vi "Winch v3.vi"() -> ()   [LabVIEW 2013]
uses:
  <vilib>/Rock Robotics/WPI/Joystick/WPI_JoystickGetSetRefNum.vi
  Robot Global Data.vi
  Globals/Useful Values.vi
  Globals/Homes.vi
  <vilib>/addons/control/pid/pid.llb/PID (DBL).vi
  Globals/Data for Dashboard.vi
  <vilib>/Utility/file.llb/Write To Spreadsheet File (DBL).vi
  <vilib>/addons/control/pid/NI_PID_pid.lvlib
panel:
  in  "Pullback Speed":dbl=-1.0
  in  "PID gains":T1={"proportional gain (Kc)"=2.75, "integral time (Ti, min)"=0.0, "derivative time (Td, min)"=0.0} {"derivative time (Td, min)" format="%.3f"; "integral time (Ti, min)" format="%.3f"; "proportional gain (Kc)" format="%.3f"}
  # "PULLBACK SPEED NEEDS\nTO BE NEGATIVE OR ELSE"
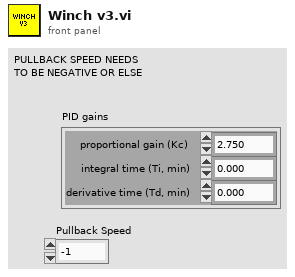
[diagram p1: front panel]
types:
  T1 = cluster{"proportional gain (Kc)":dbl, "integral time (Ti, min)":dbl, "derivative time (Td, min)":dbl}
  T2 = typedef "WPI_JoystickDevRef.ctl" = cluster{"Device":T3}
  T3 = typedef "WPI_JoystickDeviceEnum.ctl" = enum16{"USB 1", "USB 2", "USB 3", "USB 4", "Kinect 1", "Kinect 2"}
  T4 = typedef "WPI_MotorControlDeviceRef.ctl" = cluster{"DeviceStatus":errorcluster, "Type":enum16{"PWM", "CAN"}, "PWM":cluster{"Digital Module":T5, "PWM Channel":T6, "DeadBand":T7}, "CAN":cluster{"Device Number":u8, "Control Mode":T8, "Semaphore":T9, "Max Vout":dbl}, "Invert":bool, "TransformRef":T10, "InvTransformRef":T10}
  T5 = typedef "FPGA_TypedefDigitalModule.ctl" = enum16{"Digital Module 1", "Digital Module 2"}
  T6 = typedef "FPGA_DIOPWMChannel.ctl" = enum8{"PWM 1", "PWM 2", "PWM 3", "PWM 4", "PWM 5", "PWM 6", "PWM 7", "PWM 8", "PWM 9", "PWM 10", "Invalid"}
  T7 = typedef "WPI_PWMDeadband.ctl" = cluster{"Name":string, "maxPositivePwm":i32, "minPositivePwm":i32, "centerPwm":i32, "maxNegativePwm":i32, "minNegativePwm":i32, "angularRange":u16}
  T8 = typedef "WPI_CANJaguar_ControlMode.ctl" = enum8{"Percent VBus", "Current", "Speed", "Position", "Voltage"}
  T9 = typedef "Semaphore RefNum" = refnum<k1>
  T10 = typedef "WPI_PWMTransform_ConPane.ctl" = refnum<vi>
  T11 = typedef "WPI_AnalogChannelDevRef.ctl" = cluster{"DevStatus":errorcluster, "Analog Module":T12, "Analog Channel":T13}
  T12 = typedef "FPGA_TypedefAnalogModule.ctl" = enum16{"Analog Module 1", "Analog Module 2"}
  T13 = typedef "FPGA_AIChannel.ctl" = enum8{"AI 1", "AI 2", "AI 3", "AI 4", "AI 5", "AI 6", "AI 7", "AI 8", "Invalid"}
  T14 = typedef "WPI_DigitalInputDevRef.ctl" = cluster{"DevStatus":errorcluster, "DIO Channel":T15, "Digital Module":T5}
  T15 = typedef "FPGA_DIOChannel.ctl" = enum8{"DIO 1", "DIO 2", "DIO 3", "DIO 4", "DIO 5", "DIO 6", "DIO 7", "DIO 8", "DIO 9", "DIO 10", "DIO 11", "DIO 12", "DIO 13", "DIO 14", "Invalid"}
  T16 = typedef "WPI_DriverStationRobotMode2.ctl" = enum16{"Autonomous Disabled", "Autonomous Enabled", "Teleop Disabled", "Teleop Enabled", "Timeout", "Finish", "Test Disabled", "Test Enabled"}
  T17 = typedef "WPI_JoystickButtonState.ctl" = cluster{"Button 1":bool, "Button 2":bool, "Button 3":bool, "Button 4":bool, "Button 5":bool, "Button 6":bool, "Button 7":bool, "Button 8":bool, "Button 9":bool, "Button 10":bool, "Button 11":bool, "Button 12":bool}
  T18 = cluster{"axis 1 (x)":dbl, "axis 2 (y)":dbl, "axis 3 (throttle)":dbl, "axis 4":dbl, "axis 5":dbl, "axis 6":dbl}
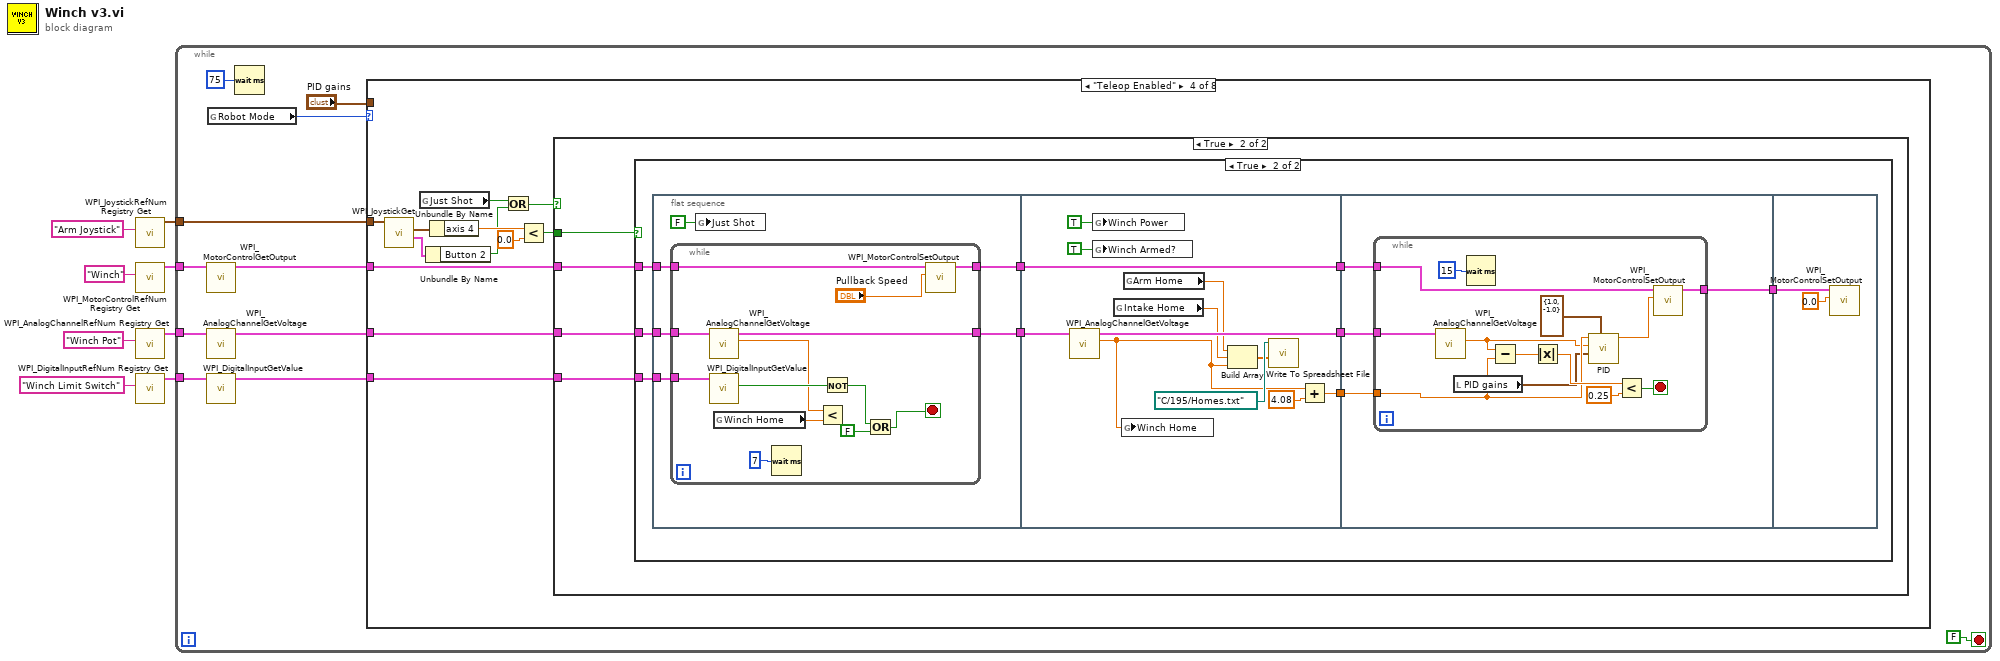
[diagram p0: block diagram]
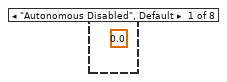
[diagram p2: hidden frame]
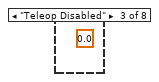
[diagram p4: hidden frame]
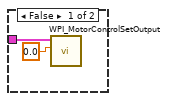
[diagram p5: hidden frame]
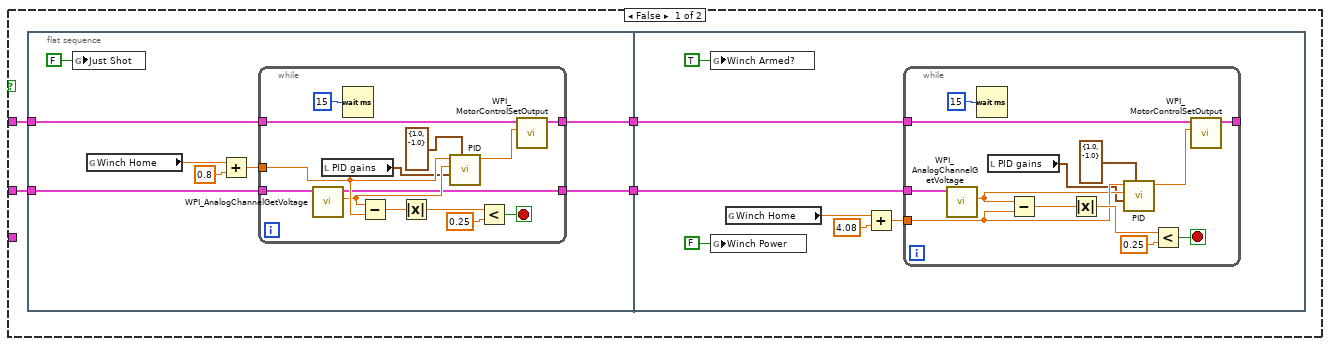
[diagram p6: hidden frame]
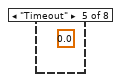
[diagram p7: hidden frame]
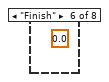
[diagram p8: hidden frame]
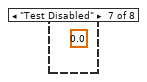
[diagram p9: hidden frame]
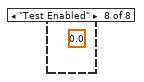
[diagram p10: hidden frame]
diagram:
  n1 = call <vilib>:"WPI_JoystickRefNum Registry Get.vi"("refnum name"="Arm Joystick") -> ("JoystickDevRef"=w3:T2)  [unwired: 9 in, 1 out]
  n2 = call <vilib>:"WPI_MotorControlRefNum Registry Get.vi"("refnum name"="Winch") -> ("MotorControlDevRef"=w5:T4)  [unwired: 9 in, 1 out]
  n3 = call <vilib>:"WPI_AnalogChannelRefNum Registry Get.vi"("refnum name"="Winch Pot") -> ("AIDeviceRef"=w8:T11)  [unwired: 9 in, 1 out]
  n4 = call <vilib>:"WPI_DigitalInputRefNum Registry Get.vi"("refnum name"="Winch Limit Switch") -> ("DigitalInputDevRef"=w2:T14)  [unwired: 9 in, 1 out]
  n5 = while {
    tunnel: w8 -> [w17]
    tunnel: w5 -> [w12]
    tunnel: w3 -> [w14]
    tunnel: w2 -> [w10]
    stop <- FALSE stop-if-true
    n6 = call <vilib>:"WPI_MotorControlGetOutput.vi"("MotorControlDevRef"=w12) -> ("MotorControlDevRef"=w11:T4)  [unwired: 8 in, 2 out]
    n7 = call <vilib>:"WPI_AnalogChannelGetVoltage.vi"("AIDeviceRef"=w17) -> ("AIDeviceRef"=w13:T11)  [unwired: 8 in, 2 out]
    n8 = call <vilib>:"WPI_DigitalInputGetValue.vi"("DigitalInputDevRef"=w10) -> ("DigitalInputDevRef"=w9:T14)  [unwired: 8 in, 2 out]
    n9 = global read "Robot Global Data.vi" "Robot Mode"() -> (w16:T16)
    n10 = Wait (ms)(milliseconds to wait=u32 75) -> ()  [unwired: 1 out]
    n11 = case shown="\"Teleop Enabled\"" w16 {
      tunnel: w11 -> [_ _ _ w28 _ _ _ _]
      tunnel: "PID gains" -> [_ _ _ _ _ _ _ _]
      tunnel: w14 -> [_ _ _ w31 _ _ _ _]
      tunnel: w9 -> [_ _ _ w29 _ _ _ _]
      tunnel: w13 -> [_ _ _ w27 _ _ _ _]
      frame "Autonomous Disabled", Default {
        (unwired) 0.0 ("Motor Output")
      }
      frame "Autonomous Enabled" {
      }
      frame "Teleop Disabled" {
        (unwired) 0.0 ("Motor Output")
      }
      frame "Teleop Enabled" {
        n12 = call <vilib>:"WPI_JoystickGet.vi"("JoystickDevRef"=w31) -> ("Buttons"=w30:T17, "Axes"=w26:T18)  [unwired: 4 in, 1 out]
        n13 = global read "Useful Values.vi" "Just Shot"() -> (w22:bool)
        n14 = Unbundle By Name(w30) -> ("Button 2"=w21:bool)
        n15 = Unbundle By Name(w26) -> ("axis 4"=w25:dbl)
        n16 = Or(x=w22, y=w21) -> (x .or. y?=w20:bool)
        n17 = Less?(x=w25, y=0.0) -> (x < y?=w23:bool)
        n18 = case shown="True" w20 {
          tunnel: w29 -> [_ w36]
          tunnel: w28 -> [w33 w37]
          tunnel: w27 -> [_ w35]
          tunnel: w23 -> [_ w34]
          frame False {
            n19 = call <vilib>:"WPI_MotorControlSetOutput.vi"("Output"=0.0, "MotorControlDevRef"=w33) -> ()  [unwired: 7 in, 3 out]
          }
          frame True {
            n20 = case shown="True" w34 {
              tunnel: w37 -> [w41 w86]
              tunnel: w36 -> [_ w85]
              tunnel: w35 -> [w40 w84]
              frame False {
                n21 = flat-sequence {
                  tunnel: w41 -> [w49]
                  tunnel: w40 -> [w48]
                  tunnel: [w44] -> w39
                  tunnel: [w43] -> w38
                  tunnel: w39 -> [w70]
                  tunnel: w38 -> [w69]
                  frame #0 {
                    n22 = global write "Useful Values.vi" "Just Shot"(FALSE ("Just Shot")) -> ()
                    n23 = global read "Homes.vi" "Winch Home"() -> (w47:dbl)
                    n24 = Add(x=w47, y=0.8) -> (x+y=w45:dbl)
                    n25 = while {
                      tunnel: w49 -> [w63]
                      tunnel: w45 -> [w56]
                      tunnel: w48 -> [w58]
                      tunnel: [w54] -> w44
                      tunnel: [w50] -> w43
                      stop <- w60 stop-if-true
                      n26 = call <vilib>:"WPI_AnalogChannelGetVoltage.vi"("AIDeviceRef"=w58) -> ("Voltage"=w55:dbl, "AIDeviceRef"=w50:T11)  [unwired: 8 in, 1 out]
                      n27 = local read "PID gains"() -> (w53:T1)
                      n28 = Wait (ms)(milliseconds to wait=u32 15) -> ()  [unwired: 1 out]
                      n29 = Subtract(x=w55, y=w56) -> (x-y=w62:dbl)
                      n30 = Absolute Value(x=w62) -> (abs(x)=w61:dbl)
                      n31 = call-poly <vilib>:"PID.vi"("output range"=cluster{"output high":dbl, "output low":dbl} {"output high"=1.0, "output low"=-1.0}, "PID gains"=w53, "process variable"=w55, "setpoint"=w56) -> ("output"=w51:dbl)  [unwired: 6 in, 1 out]
                      n32 = Less?(x=w61, y=0.25) -> (x < y?=w60:bool)
                      n33 = call <vilib>:"WPI_MotorControlSetOutput.vi"("Output"=w51, "MotorControlDevRef"=w63) -> ("MotorControlDevRef"=w54:T4)  [unwired: 7 in, 2 out]
                    }
                  }
                  frame #1 {
                    n34 = global write "Data for Dashboard.vi" "Winch Armed?"(TRUE ("Loaded")) -> ()
                    n35 = global write "Data for Dashboard.vi" "Winch Power"(FALSE ("Loaded")) -> ()
                    n36 = global read "Homes.vi" "Winch Home"() -> (w68:dbl)
                    n37 = Add(x=w68, y=4.08) -> (x+y=w66:dbl)
                    n38 = while {
                      tunnel: w70 -> [w83]
                      tunnel: w66 -> [w76]
                      tunnel: w69 -> [w78]
                      tunnel: [w74] -> _
                      stop <- w80 stop-if-true
                      n39 = call <vilib>:"WPI_AnalogChannelGetVoltage.vi"("AIDeviceRef"=w78) -> ("Voltage"=w75:dbl)  [unwired: 8 in, 2 out]
                      n40 = Wait (ms)(milliseconds to wait=u32 15) -> ()  [unwired: 1 out]
                      n41 = local read "PID gains"() -> (w73:T1)
                      n42 = Subtract(x=w75, y=w76) -> (x-y=w82:dbl)
                      n43 = Absolute Value(x=w82) -> (abs(x)=w81:dbl)
                      n44 = call-poly <vilib>:"PID.vi"("output range"=cluster{"output high":dbl, "output low":dbl} {"output high"=1.0, "output low"=-1.0}, "PID gains"=w73, "process variable"=w75, "setpoint"=w76) -> ("output"=w71:dbl)  [unwired: 6 in, 1 out]
                      n45 = Less?(x=w81, y=0.25) -> (x < y?=w80:bool)
                      n46 = call <vilib>:"WPI_MotorControlSetOutput.vi"("Output"=w71, "MotorControlDevRef"=w83) -> ("MotorControlDevRef"=w74:T4)  [unwired: 7 in, 2 out]
                    }
                  }
                }
              }
              frame True {
                n47 = flat-sequence {
                  tunnel: w85 -> [w98]
                  tunnel: w86 -> [w97]
                  tunnel: [w96] -> w92
                  tunnel: [w93] -> w91
                  tunnel: w84 -> [w94]
                  tunnel: w92 -> [w123]
                  tunnel: [w123] -> w90
                  tunnel: [w122] -> w89
                  tunnel: w91 -> [w121]
                  tunnel: [w120] -> w88
                  tunnel: w90 -> [w127]
                  tunnel: w89 -> [w125]
                  tunnel: [w124] -> w87
                  tunnel: w88 -> [w126]
                  tunnel: w87 -> [w142]
                  frame #0 {
                    n48 = while {
                      tunnel: w98 -> [w111]
                      tunnel: w97 -> [w107]
                      tunnel: [w106] -> w96
                      tunnel: w94 -> [w105]
                      tunnel: [w104] -> w93
                      stop <- w101 stop-if-true
                      n49 = call <vilib>:"WPI_AnalogChannelGetVoltage.vi"("AIDeviceRef"=w105) -> ("Voltage"=w103:dbl, "AIDeviceRef"=w104:T11)  [unwired: 8 in, 1 out]
                      n50 = call <vilib>:"WPI_DigitalInputGetValue.vi"("DigitalInputDevRef"=w111) -> ("Value"=w110:bool)  [unwired: 8 in, 2 out]
                      n51 = global read "Homes.vi" "Winch Home"() -> (w102:dbl)
                      n52 = Wait (ms)(milliseconds to wait=u32 7) -> ()  [unwired: 1 out]
                      n53 = Less?(x=w103, y=w102) -> ()  [unwired: 1 out]
                      n54 = Not(x=w110) -> (.not. x?=w100:bool)
                      n55 = Or(x=w100, y=FALSE) -> (x .or. y?=w101:bool)
                      n56 = call <vilib>:"WPI_MotorControlSetOutput.vi"("Output"="Pullback Speed", "MotorControlDevRef"=w107) -> ("MotorControlDevRef"=w106:T4)  [unwired: 7 in, 2 out]
                    }
                    n57 = global write "Useful Values.vi" "Just Shot"(FALSE ("Just Shot")) -> ()
                  }
                  frame #1 {
                    n58 = call <vilib>:"WPI_AnalogChannelGetVoltage.vi"("AIDeviceRef"=w121) -> ("Voltage"=w114:dbl, "AIDeviceRef"=w122:T11)  [unwired: 8 in, 1 out]
                    n59 = global write "Data for Dashboard.vi" "Winch Power"(TRUE ("Loaded")) -> ()
                    n60 = global write "Data for Dashboard.vi" "Winch Armed?"(TRUE ("Loaded")) -> ()
                    n61 = global read "Homes.vi" "Intake Home"() -> (w115:dbl)
                    n62 = global write "Homes.vi" "Winch Home"(w114) -> ()
                    n63 = global read "Homes.vi" "Arm Home"() -> (w117:dbl)
                    n64 = Build Array(w117, w115, w114) -> (w116:dbl[])
                    n65 = call-poly <vilib>:"Write To Spreadsheet File.vi"("1D data"=w116, "file path (dialog if empty)"=path "C:/195/Homes.txt") -> ()  [unwired: 6 in, 1 out]
                    n66 = Add(x=w114, y=4.08) -> (x+y=w120:dbl)
                  }
                  frame #2 {
                    n67 = while {
                      tunnel: w127 -> [w140]
                      tunnel: w126 -> [w133]
                      tunnel: w125 -> [w135]
                      tunnel: [w131] -> w124
                      stop <- w137 stop-if-true
                      n68 = call <vilib>:"WPI_AnalogChannelGetVoltage.vi"("AIDeviceRef"=w135) -> ("Voltage"=w132:dbl)  [unwired: 8 in, 2 out]
                      n69 = local read "PID gains"() -> (w130:T1)
                      n70 = Wait (ms)(milliseconds to wait=u32 15) -> ()  [unwired: 1 out]
                      n71 = Subtract(x=w132, y=w133) -> (x-y=w139:dbl)
                      n72 = Absolute Value(x=w139) -> (abs(x)=w138:dbl)
                      n73 = call-poly <vilib>:"PID.vi"("output range"=cluster{"output high":dbl, "output low":dbl} {"output high"=1.0, "output low"=-1.0}, "PID gains"=w130, "process variable"=w132, "setpoint"=w133) -> ("output"=w128:dbl)  [unwired: 6 in, 1 out]
                      n74 = Less?(x=w138, y=0.25) -> (x < y?=w137:bool)
                      n75 = call <vilib>:"WPI_MotorControlSetOutput.vi"("Output"=w128, "MotorControlDevRef"=w140) -> ("MotorControlDevRef"=w131:T4)  [unwired: 7 in, 2 out]
                    }
                  }
                  frame #3 {
                    n76 = call <vilib>:"WPI_MotorControlSetOutput.vi"("Output"=0.0, "MotorControlDevRef"=w142) -> ()  [unwired: 7 in, 3 out]
                  }
                }
              }
            }
          }
        }
      }
      frame "Timeout" {
        (unwired) 0.0 ("Motor Output")
      }
      frame "Finish" {
        (unwired) 0.0 ("Motor Output")
      }
      frame "Test Disabled" {
        (unwired) 0.0 ("Motor Output")
      }
      frame "Test Enabled" {
        (unwired) 0.0 ("Motor Output")
      }
    }
  }
